vi "PID for position.vi"(7 "output range":cluster{"output high":dbl, "output low":dbl}[](array[cluster])=[{"output high"=100.0, "output low"=-100.0}] {"output low" format="%.2f"; "output high" format="%.2f"}, 9 "PID gains":T2(array[cluster])=[{"proportional gain (Kc)"=1.0, "integral time (Ti, min)"=0.01, "derivative time (Td, min)"=0.0}] {"derivative time (Td, min)" format="%.3f"; "integral time (Ti, min)" format="%.3f"; "proportional gain (Kc)" format="%.3f"}, 10 "mes force":dbl[](array[numeric]), 11 "ref force":dbl[](array[numeric])) -> (1 "output cluster":T1, 3 "PID output":dbl[](array[numeric]))   [LabVIEW 2021]
uses:
  <vilib>/addons/control/pid/pid.llb/PID (DBL Array).vi
  <vilib>/addons/control/pid/NI_PID_pid.lvlib
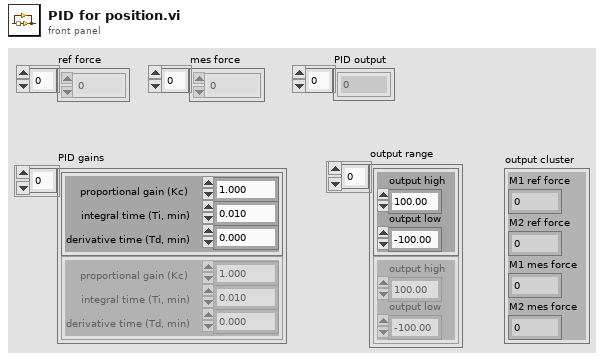
[diagram p1: front panel]
types:
  T1 = cluster{"M1 ref force":dbl, "M2 ref force":dbl, "M1 mes force":dbl, "M2 mes force":dbl}
  T2 = cluster{"proportional gain (Kc)":dbl, "integral time (Ti, min)":dbl, "derivative time (Td, min)":dbl}[]
  T3 = cluster{"Set Point (N)":dbl, "Set Point (N)":dbl, "Filtered x":dbl, "Filtered x":dbl}
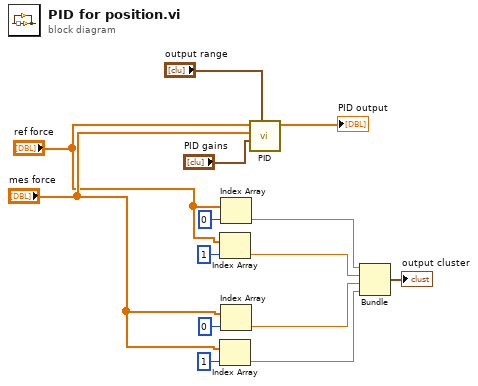
[diagram p0: block diagram]
diagram:
  n1 = Index Array(array="ref force", index=1) -> (element=w4:dbl)
  n2 = Index Array(array="mes force", index=1) -> (element=w2:dbl)
  n3 = Index Array(array="ref force", index=0) -> (element=w5:dbl)
  n4 = Index Array(array="mes force", index=0) -> (element=w3:dbl)
  n5 = call-poly <vilib>:"PID.vi"("output range"="output range", "PID gains"="PID gains", "process variable"="mes force", "setpoint"="ref force") -> ("output"=→"PID output":dbl[])  [unwired: 6 in, 1 out]
  n6 = Bundle("Set Point (N)"=w5, "Set Point (N)"=w4, "Filtered x"=w3, "Filtered x"=w2) -> (→"output cluster":T3)  [unwired: 1 in]
